vi "MultiTauCorrelation.vi"(6 "zero lag +":i32=1, 9 "AC final pts":i64=64, 10 "counts":dbl[](array[numeric]), 11 "First Call":i32=2) -> (2 "Mean of  Bins":dbl format="%0.2f", 3 "Data out":dbl[][](array[numeric]))   [LabVIEW 2022 SP3]
uses:
  <vilib>/Analysis/baseanly.llb/Mean (DBL).vi
  <vilib>/Analysis/NI_AALBase.lvlib
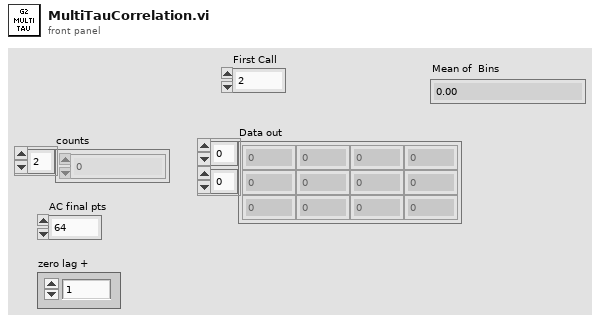
[diagram p1: front panel]
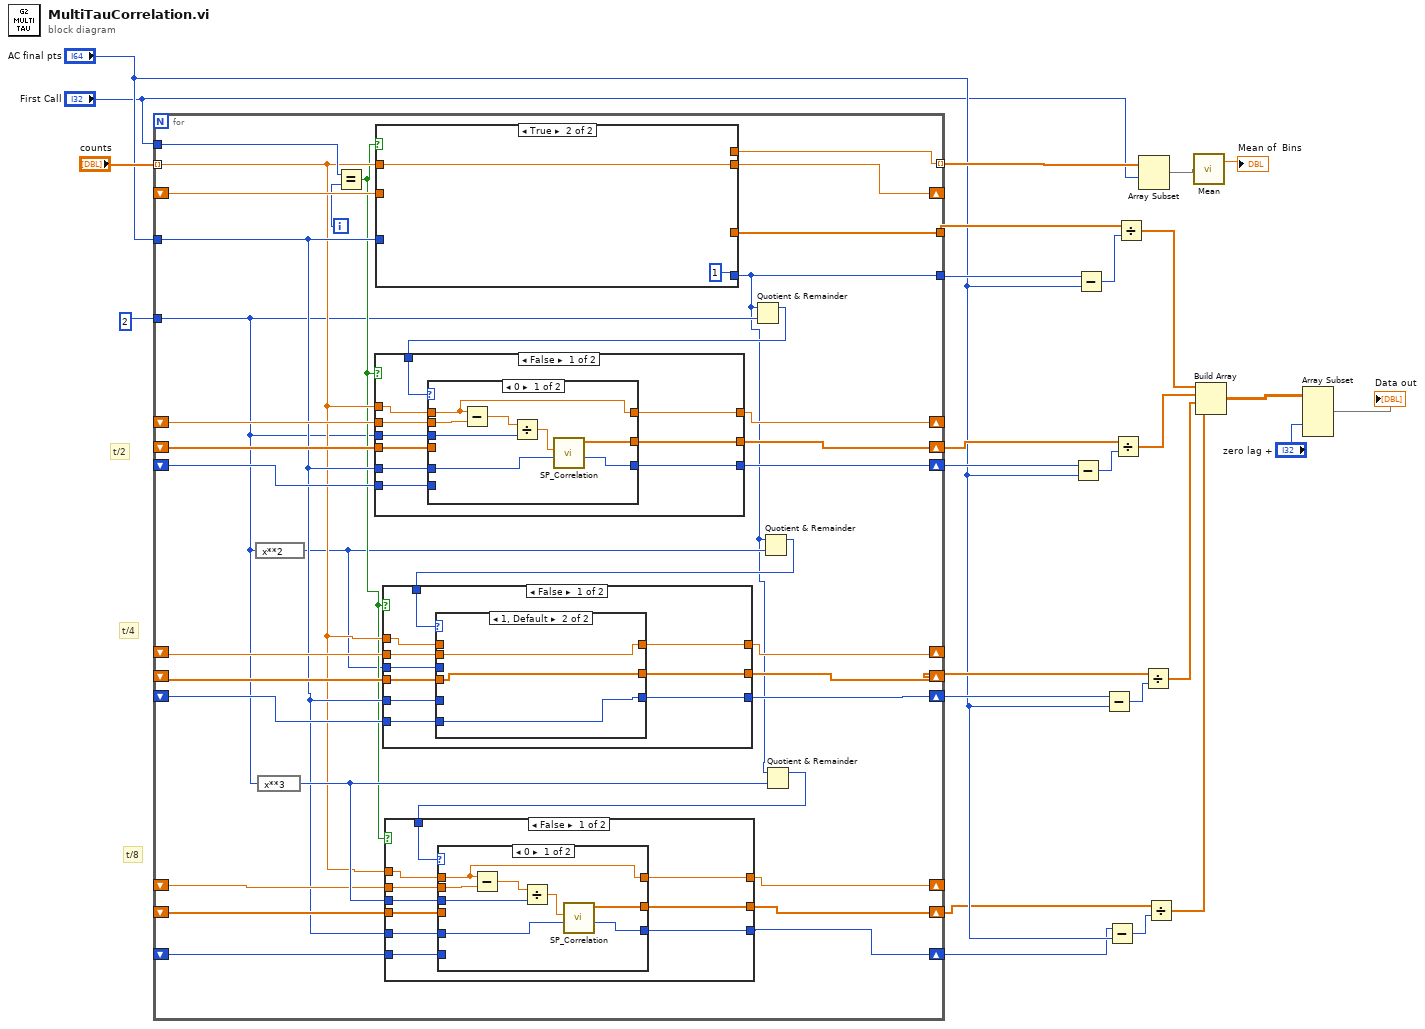
[diagram p0: block diagram]
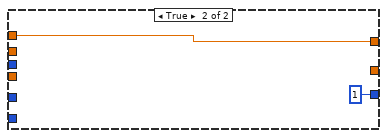
[diagram p3: hidden frame]
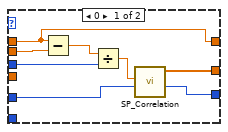
[diagram p4: hidden frame]
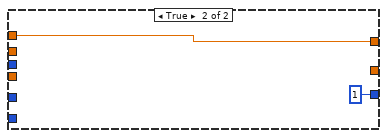
[diagram p5: hidden frame]
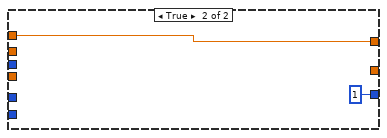
[diagram p7: hidden frame]
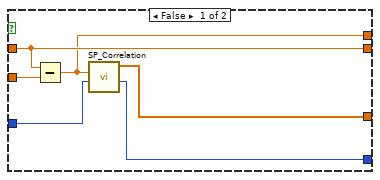
[diagram p8: hidden frame]
diagram:
  # "t/8"
  # "t/4"
  # "t/2"
  n1 = for {
    tunnel: "counts" -> [w36] mode=indexing
    tunnel: "AC final pts" -> [w37]
    tunnel: [w60] -> w25
    shift-right: [w42] -> _
    shift-left: _ -> [w59]
    tunnel: "First Call" -> [w54]
    tunnel: [w28] -> w24
    tunnel: 2 -> [w33]
    shift-right: [w56] -> _
    shift-left: _ -> [w55]
    shift-right: [w58] -> w22
    shift-left: _ -> [w52]
    shift-right: [w50] -> _
    shift-left: _ -> [w48]
    shift-right: [w49] -> w18
    shift-left: _ -> [w47]
    shift-right: [w45] -> w21
    shift-left: _ -> [w44]
    shift-right: [w46] -> w17
    shift-left: _ -> [w43]
    tunnel: [w27] -> w11 mode=indexing
    shift-right: [w32] -> _
    shift-left: _ -> [w40]
    shift-right: [w31] -> w5
    shift-left: _ -> [w38]
    shift-right: [w30] -> w4
    shift-left: _ -> [w39]
    i -> [w53]
    n2 = expression code="x**2"(w33) -> (w34:i32)
    n3 = expression code="x**3"(w33) -> (w41:i32)
    n4 = Equal?(x=w54, y=w53) -> (x = y?=w35:bool)
    n5 = case shown="True" w35 {
      tunnel: w37 -> [w135 _]
      tunnel: [w134 _] -> w60
      tunnel: [w132 1 ("interation")] -> w28
      tunnel: w59 -> [w133 _]
      tunnel: w36 -> [w131 w137]
      tunnel: [w131 w137] -> w42
      tunnel: [w130 _] -> w27
      frame False {
        n6 = Subtract(x=w131, y=w133) -> (x-y=w130:dbl)
        n7 = call "SP_Correlation.vi"("Tau Number"=w135, "New Count"=w130) -> ("interation"=w132:i64, "Cross Corr"=w134:dbl[])  [unwired: 8 in]
      }
      frame True {
      }
    }
    n8 = Quotient & Remainder(x=w28, y=w33) -> (x-y*floor(x/y)=w57:i64)  [unwired: 1 out]
    n9 = case shown="False" w35 {
      tunnel: w37 -> [w116 _]
      tunnel: [w115 _] -> w58
      tunnel: [w112 1 ("interation")] -> w45
      tunnel: w55 -> [w114 _]
      tunnel: w36 -> [w113 w129]
      tunnel: w57 -> [w111 _]
      tunnel: [w110 w129] -> w56
      tunnel: w33 -> [w109 _]
      tunnel: w52 -> [w108 _]
      tunnel: w44 -> [w107 _]
      frame False {
        n10 = case shown="0" w111 {
          tunnel: w116 -> [w124 _]
          tunnel: [w123 w127] -> w115
          tunnel: w114 -> [w122 w125]
          tunnel: w113 -> [w120 _]
          tunnel: [w121 w126] -> w112
          tunnel: [w120 w125] -> w110
          tunnel: w109 -> [w119 _]
          tunnel: w108 -> [_ w127]
          tunnel: w107 -> [_ w126]
          frame 0 {
            n11 = Subtract(x=w120, y=w122) -> (x-y=w118:dbl)
            n12 = Divide(x=w118, y=w119) -> (x/y=w117:dbl)
            n13 = call "SP_Correlation.vi"("Tau Number"=w124, "New Count"=w117) -> ("interation"=w121:i64, "Cross Corr"=w123:dbl[])  [unwired: 8 in]
          }
          frame 1, Default {
          }
        }
      }
      frame True {
      }
    }
    n14 = Quotient & Remainder(x=w28, y=w34) -> (x-y*floor(x/y)=w51:i64)  [unwired: 1 out]
    n15 = case shown="False" w35 {
      tunnel: w37 -> [w93 _]
      tunnel: [w92 _] -> w49
      tunnel: [w89 1 ("interation")] -> w46
      tunnel: w48 -> [w91 _]
      tunnel: w36 -> [w90 w106]
      tunnel: w51 -> [w88 _]
      tunnel: [w87 w106] -> w50
      tunnel: w34 -> [w86 _]
      tunnel: w47 -> [w85 _]
      tunnel: w43 -> [w84 _]
      frame False {
        n16 = case shown="1, Default" w88 {
          tunnel: w93 -> [w101 _]
          tunnel: [w100 w104] -> w92
          tunnel: w91 -> [w99 w102]
          tunnel: w90 -> [w97 _]
          tunnel: [w98 w103] -> w89
          tunnel: [w97 w102] -> w87
          tunnel: w86 -> [w96 _]
          tunnel: w85 -> [_ w104]
          tunnel: w84 -> [_ w103]
          frame 0 {
            n17 = Subtract(x=w97, y=w99) -> (x-y=w95:dbl)
            n18 = Divide(x=w95, y=w96) -> (x/y=w94:dbl)
            n19 = call "SP_Correlation.vi"("Tau Number"=w101, "New Count"=w94) -> ("interation"=w98:i64, "Cross Corr"=w100:dbl[])  [unwired: 8 in]
          }
          frame 1, Default {
          }
        }
      }
      frame True {
      }
    }
    n20 = Quotient & Remainder(x=w28, y=w41) -> (x-y*floor(x/y)=w29:i64)  [unwired: 1 out]
    n21 = case shown="False" w35 {
      tunnel: w37 -> [w70 _]
      tunnel: [w69 _] -> w30
      tunnel: [w66 1 ("interation")] -> w31
      tunnel: w40 -> [w68 _]
      tunnel: w36 -> [w67 w83]
      tunnel: w29 -> [w65 _]
      tunnel: [w64 w83] -> w32
      tunnel: w41 -> [w63 _]
      tunnel: w39 -> [w62 _]
      tunnel: w38 -> [w61 _]
      frame False {
        n22 = case shown="0" w65 {
          tunnel: w70 -> [w78 _]
          tunnel: [w77 w81] -> w69
          tunnel: w68 -> [w76 w79]
          tunnel: w67 -> [w74 _]
          tunnel: [w75 w80] -> w66
          tunnel: [w74 w79] -> w64
          tunnel: w63 -> [w73 _]
          tunnel: w62 -> [_ w81]
          tunnel: w61 -> [_ w80]
          frame 0 {
            n23 = Subtract(x=w74, y=w76) -> (x-y=w72:dbl)
            n24 = Divide(x=w72, y=w73) -> (x/y=w71:dbl)
            n25 = call "SP_Correlation.vi"("Tau Number"=w78, "New Count"=w71) -> ("interation"=w75:i64, "Cross Corr"=w77:dbl[])  [unwired: 8 in]
          }
          frame 1, Default {
          }
        }
      }
      frame True {
      }
    }
  }
  n26 = Subtract(x=w21, y="AC final pts") -> (x-y=w23:i64)
  n27 = Subtract(x=w24, y="AC final pts") -> (x-y=w26:i64)
  n28 = Subtract(x=w17, y="AC final pts") -> (x-y=w19:i64)
  n29 = Subtract(x=w5, y="AC final pts") -> (x-y=w7:i64)
  n30 = Divide(x=w22, y=w23) -> (x/y=w15:dbl[])
  n31 = Divide(x=w25, y=w26) -> (x/y=w16:dbl[])
  n32 = Array Subset(array=w11, index="First Call") -> (w9:dbl[])  [unwired: 1 in]
  n33 = Divide(x=w18, y=w19) -> (x/y=w10:dbl[])
  n34 = Divide(x=w4, y=w7) -> (x/y=w3:dbl[])
  n35 = call-poly <vilib>:"Mean.vi"("X"=w9) -> ("mean"=→"Mean of  Bins":dbl)  [unwired: 1 out]
  n36 = Build Array(w16, w15, w10, w3) -> (w14:dbl[][])
  n37 = Array Subset(array=w14, index (col)="zero lag +") -> (→"Data out":dbl[][])  [unwired: 3 in]
